vi "Start Game.vi"(11 "SB App in":refnum<class "SB App.lvclass">) -> (3 "SB App out":refnum<class "SB App.lvclass">)   [LabVIEW 2020, in "SB App.lvlib" / "SB App.lvclass"]
uses:
  SB App.lvclass
  SB App.lvclass/SB App.ctl
  SquareBattle/Game/Game.lvclass
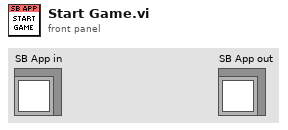
[diagram p1: front panel]
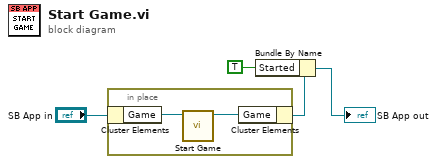
[diagram p0: block diagram]
diagram:
  n1 = in-place {
    n2 = in-place-cluster #1("SB App in") -> ("Game"=w6:refnum<class "Game.lvclass">)
    n3 = call "Start Game.vi"("Game in"=w6) -> ("Game out"=w5:refnum<class "Game.lvclass">)  [unwired: 9 in, 1 out]
    n4 = in-place-cluster #1("Game"=w5) -> (w3:refnum<class "SB App.lvclass">)
  }
  n5 = Bundle By Name(cluster=w3, "Started"=TRUE ("Running")) -> (→"SB App out":refnum<class "SB App.lvclass">)
